vi "Create Control.vi"(8 "error in (no error)":errorcluster, 10 "Variant in":variant, 11 "Path to save control":path) -> (0 "error out":errorcluster)   [LabVIEW 2017, in "Advanced Variant Tools.lvlib" / "Control Scripting.lvlib"]
uses:
  Control Scripting.lvlib
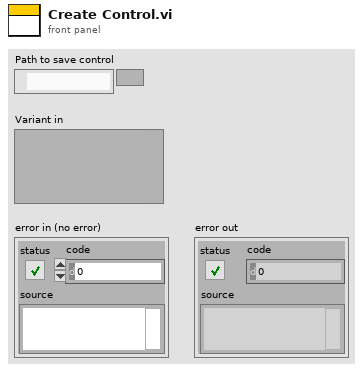
[diagram p1: front panel]
types:
  T1 = enum32{"invalid VI type", "Standard VI", "Control VI", "Global VI", "Polymorphic VI", "Configuration VI", "SubSystem", "Facade VI", "Method VI", "Statechart Diagram VI"}
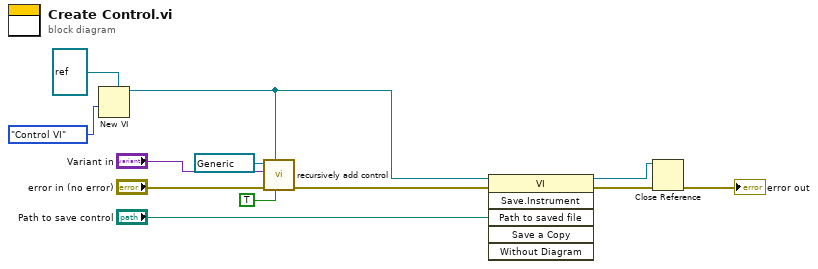
[diagram p0: block diagram]
diagram:
  n1 = New VI(5:refnum<vi> refnum ("type specifier VI Refnum (for type only)"), 9:T1."Control VI" ("vi type (standard vi)")) -> (3:w3:refnum<vi>)  [unwired: 5 in, 1 out]
  n2 = call "recursively add control.vi"("use VI refnum"=TRUE, "vi refnum"=w3, "error in (no error)"="error in (no error)", "Variant in"="Variant in", "object refnum"=refnum<vi> refnum) -> ("error out"=w9:errorcluster)  [unwired: 6 in]
  n3 = invoke class="VI" method="Save.Instrument"(reference=w3, error in=w9, "Path to saved file"="Path to save control") -> (reference out=w4:refnum<vi>, error out=w8:errorcluster)  [unwired: 3 in, 4 out]
  n4 = Close Reference(reference=w4, error in (no error)=w8) -> (error out=→"error out":errorcluster)
